vi "Car_Position.vi"(3 "error in (no error)":errorcluster, 4 "Car Wash Indicators":refnum<vi>, 5 "Data":variant, 6 "System data in":T2) -> (0 "error out":errorcluster, 1 "State":T1, 2 "System data out":T2)   [LabVIEW 2023]
uses:
  Controls/System_Data.ctl
  Controls/Wash Options.ctl
  Controls/State.ctl
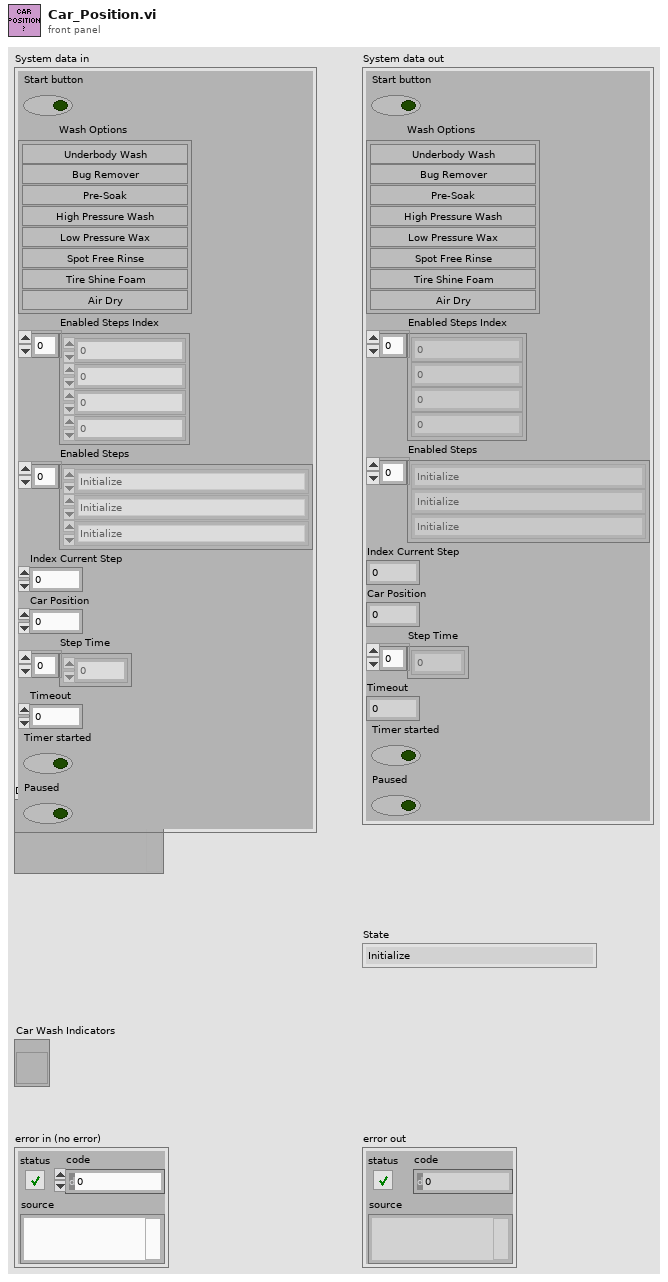
[diagram p1: front panel]
types:
  T1 = typedef "State.ctl" = enum16{"Initialize", "Wait for Something", "Step Completed", "Save Wash Options", "Start Process", "Car Position", "Order Steps to follow", "Underbody Wash", "Bug Remover", "Pre-Soak", "High Pressure Wash", "Low Pressure Wax", "Spot Free Rinse", "Tire Shine Foam", "Air Dry", "Vehicle out of position", "Exit", "Process Complete", "Stop Application"}
  T2 = typedef "System_Data.ctl" = cluster{"Start button":bool, "Wash Options":T3, "Enabled Steps Index":i32[], "Enabled Steps ":T1[], "Index Current Step":i32, "Car Position":u8, "Step Time":dbl[], "Timeout":i32, "Timer started":bool, "Paused":bool}
  T3 = typedef "Wash Options.ctl" = cluster{"Underbody Wash":bool, "Bug Remover":bool, "Pre-Soak":bool, "High Pressure Wash":bool, "Low Pressure Wax":bool, "Spot Free Rinse":bool, "Tire Shine Foam":bool, "Air Dry":bool}
  T4 = typedef "Car Wash Indicators.ctl" = cluster{"Under Body Wash":bool, "Bug Remover":bool, "Pre-Soak":bool, "High Pressure Wash":bool, "Low Pressure Wax":bool, "Spot Free Rinse":bool, "Tire Shine Foam":bool, "Air Dry":bool, "Vehicle Out of Position":bool}
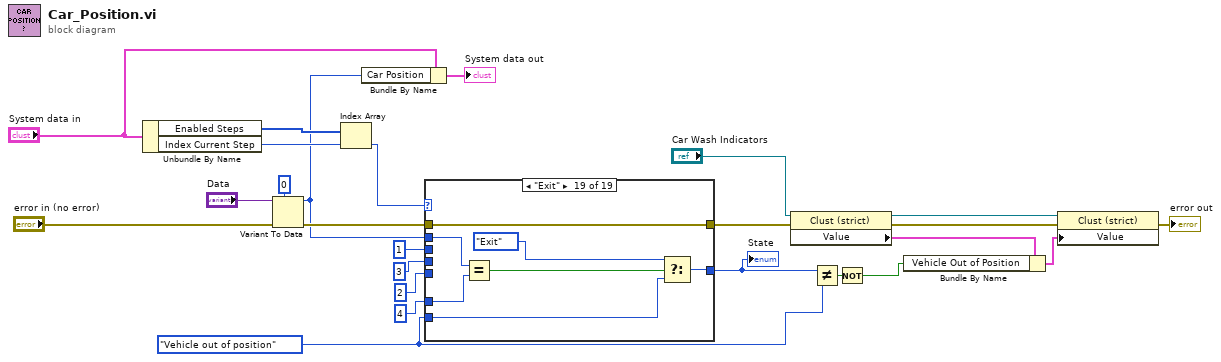
[diagram p0: block diagram]
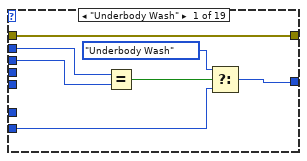
[diagram p2: hidden frame]
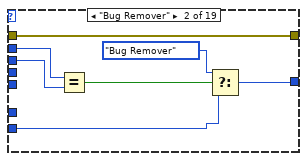
[diagram p3: hidden frame]
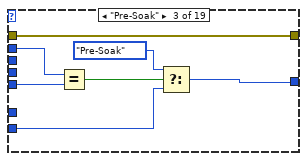
[diagram p4: hidden frame]
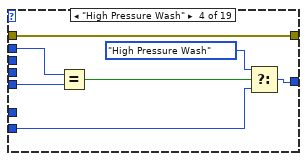
[diagram p5: hidden frame]
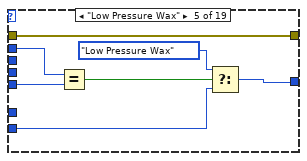
[diagram p6: hidden frame]
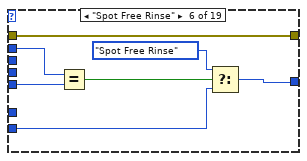
[diagram p7: hidden frame]
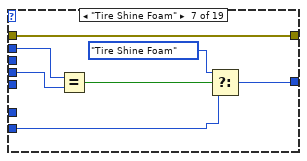
[diagram p8: hidden frame]
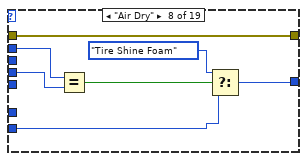
[diagram p9: hidden frame]
diagram:
  w10 = State."Vehicle out of position" ("State")
  n1 = Unbundle By Name("System data in") -> ("Enabled Steps"=w23:T1[], "Index Current Step"=w22:i32)
  n2 = Variant To Data(error in="error in (no error)", type=u8 0, Variant="Data") -> (data=w19:u8, error out=w20:errorcluster)
  n3 = Index Array(array=w23, index=w22) -> (element=w21:T1)
  n4 = Bundle By Name(cluster="System data in", "Car Position"=w19) -> (→"System data out":T2)
  n5 = case shown="\"Exit\"" w21 {
    tunnel: w20 -> [w32 w39 w46 w53 w60 w67 w74 w81 w82 w83 w84 w85 w86 w87 w88 w89 w90 w91 w98]
    tunnel: [w32 w39 w46 w53 w60 w67 w74 w81 w82 w83 w84 w85 w86 w87 w88 w89 w90 w91 w98] -> w13
    tunnel: w19 -> [w31 w36 w43 w49 w55 w63 w71 w77 _ _ _ _ _ _ _ _ _ _ w96]
    tunnel: u8 1 -> [w30 w35 _ _ _ _ _ _ _ _ _ _ _ _ _ _ _ _ _]
    tunnel: [w27 w34 w42 w50 w57 w64 w70 w78 _ _ _ _ _ _ _ _ _ _ w94] -> w11
    tunnel: u8 2 -> [_ _ w41 w48 w56 w62 _ _ _ _ _ _ _ _ _ _ _ _ _]
    tunnel: u8 3 -> [_ _ _ _ _ _ w69 w76 _ _ _ _ _ _ _ _ _ _ _]
    tunnel: w10 -> [w26 w33 w40 w47 w54 w61 w68 w75 _ _ _ _ _ _ _ _ _ _ w92]
    tunnel: u8 4 -> [_ _ _ _ _ _ _ _ _ _ _ _ _ _ _ _ _ _ w97]
    frame "Underbody Wash" {
      n6 = Equal?(x=w31, y=w30) -> (x = y?=w29:bool)
      n7 = Select(t=State."Underbody Wash" ("State"), s=w29, f=w26) -> (s? t:f=w27:T1)
    }
    frame "Bug Remover" {
      n8 = Equal?(x=w36, y=w35) -> (x = y?=w38:bool)
      n9 = Select(t=State."Bug Remover" ("State"), s=w38, f=w33) -> (s? t:f=w34:T1)
    }
    frame "Pre-Soak" {
      n10 = Equal?(x=w43, y=w41) -> (x = y?=w45:bool)
      n11 = Select(t=State."Pre-Soak" ("State"), s=w45, f=w40) -> (s? t:f=w42:T1)
    }
    frame "High Pressure Wash" {
      n12 = Equal?(x=w49, y=w48) -> (x = y?=w52:bool)
      n13 = Select(t=State."High Pressure Wash" ("State"), s=w52, f=w47) -> (s? t:f=w50:T1)
    }
    frame "Low Pressure Wax" {
      n14 = Equal?(x=w55, y=w56) -> (x = y?=w59:bool)
      n15 = Select(t=State."Low Pressure Wax" ("State"), s=w59, f=w54) -> (s? t:f=w57:T1)
    }
    frame "Spot Free Rinse" {
      n16 = Equal?(x=w63, y=w62) -> (x = y?=w66:bool)
      n17 = Select(t=State."Spot Free Rinse" ("State"), s=w66, f=w61) -> (s? t:f=w64:T1)
    }
    frame "Tire Shine Foam" {
      n18 = Equal?(x=w71, y=w69) -> (x = y?=w73:bool)
      n19 = Select(t=State."Tire Shine Foam" ("State"), s=w73, f=w68) -> (s? t:f=w70:T1)
    }
    frame "Air Dry" {
      n20 = Equal?(x=w77, y=w76) -> (x = y?=w80:bool)
      n21 = Select(t=State."Tire Shine Foam" ("State"), s=w80, f=w75) -> (s? t:f=w78:T1)
    }
    frame "Vehicle out of position" {
    }
    frame "Process Complete" {
    }
    frame "Stop Application" {
    }
    frame "Order Steps to follow" {
    }
    frame "Car Position" {
    }
    frame "Start Process" {
    }
    frame "Save Wash Options" {
    }
    frame "Step Completed" {
    }
    frame "Wait for Something" {
    }
    frame "Initialize" {
    }
    frame "Exit" {
      n22 = Equal?(x=w96, y=w97) -> (x = y?=w95:bool)
      n23 = Select(t=State."Exit" ("State"), s=w95, f=w92) -> (s? t:f=w94:T1)
    }
  }
  "State" <- w11
  n24 = property class="Clust (strict)"(reference="Car Wash Indicators", error in=w13) -> (reference out=w6:refnum<vi>, error out=w9:errorcluster, "Value"=w5:T4)
  n25 = Not Equal?(x=w11, y=w10) -> (x != y?=w3:bool)
  n26 = Not(x=w3) -> (.not. x?=w2:bool)
  n27 = Bundle By Name(cluster=w5, "Vehicle Out of Position"=w2) -> (w4:T4)
  n28 = property class="Clust (strict)"(reference=w6, error in=w9, "Value"=w4) -> (error out=→"error out":errorcluster)  [unwired: 1 out]
